vi "BaseConfigure.vi"(8 "error in (no error)":errorcluster, 11 "ChromaAcLoad in":refnum<class "ChromaAcLoad.lvclass">) -> (0 "error out":errorcluster, 3 "ChromaAcLoad out":refnum<class "ChromaAcLoad.lvclass">)   [LabVIEW 2014, in "AcPwrPlugins.lvlib" / "ChromaAcLoad.lvclass"]
uses:
  ChromaAcLoad.lvclass
  AcPwrBaseClass/AcPwrBase.lvclass/AcPwrBase.ctl
  ChromaAcLoad.lvclass/ChromaAcLoad.ctl
  AcPwrBaseClass/Accessors/Read BaseConfig.vi
  Accessors/Read Loads.vi
  AcPwrBaseClass/Accessors/Write BaseConfig.vi
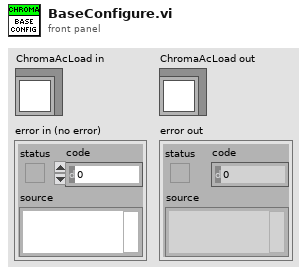
[diagram p1: front panel]
types:
  T1 = typedef "AcPwrPlugins.lvlib/AcPwrBase.lvclass/BaseConfig.ctl" = cluster{"Frequency":dbl, "FrequencyRange":dbl[], "Phases":T2[]}
  T2 = typedef "AcPwrPlugins.lvlib/AcPwrBase.lvclass/Phase.ctl" = cluster{"Enabled":bool, "VoltageLevel":dbl, "Waveform":string, "Name":string, "VoltageRange":dbl[], "CurrentLimit":dbl, "Handle":string, "Connected":bool}
  T3 = typedef "AcPwrPlugins.lvlib/ChromaAcLoad.lvclass/Load.ctl" = cluster{"AC/DC":bool, "Mode":enum16{"CC", "CP", "CR", "CV", "RLC", "RLC CP", "Inrush", "Rectified"}, "LC":cluster{"Capacitance":dbl, "Inductance":dbl, "RL":dbl, "RS":dbl}, "Resistance":dbl, "LoadSettings":T4, "Wave":enum16{""}, "LineSync":bool, "LoadShortCircuited":bool, "Slew":cluster{"RiseSlewRate":dbl, "FallSlewRate":dbl}, "Timing":cluster{"TimingOn":enum16{""}, "Hours":u32, "Minutes":u32, "Seconds":dbl, "CutoffVoltage":dbl}}
  T4 = typedef "AcPwrPlugins.lvlib/ChromaAcLoad.lvclass/LoadSettings.ctl" = cluster{"CrestFactor":dbl, "PowerFactor":dbl, "PowerLoading":dbl, "IpeakMax":dbl, "Priority":enum16{"Off", "Hold Up", "Transfer"}}
  T5 = enum16{"CC", "CP", "CR", "CV", "RLC", "RLC CP", "Inrush", "Rectified"}
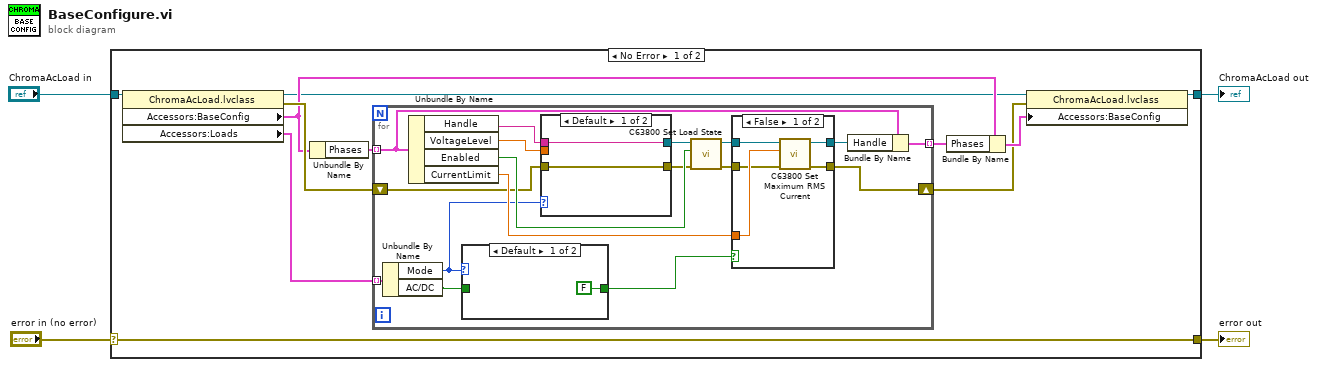
[diagram p0: block diagram]
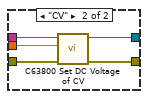
[diagram p2: hidden frame]
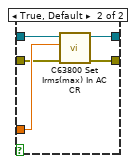
[diagram p3: hidden frame]
diagram:
  n1 = case shown="No Error" "error in (no error)" {
    selector: "error in (no error)" -> [w12 w52]
    tunnel: "ChromaAcLoad in" -> [w15 w53]
    tunnel: [w8 w53] -> w3
    tunnel: [w12 w52] -> w1
    frame No Error {
      n2 = property class="ChromaAcLoad.lvclass"(reference=w15) -> (reference out=w7:refnum<class "ChromaAcLoad.lvclass">, error out=w13:errorcluster, "Accessors:BaseConfig"=w10:T1, "Accessors:Loads"=w11:T3[])  [unwired: 1 in]
      n3 = Unbundle By Name(w10) -> ("Phases"=w14:T2[])
      n4 = for {
        tunnel: w14 -> [w25] mode=indexing
        tunnel: w11 -> [w31] mode=indexing
        tunnel: [w24] -> w9 mode=indexing
        shift-right: [w22] -> w5
        shift-left: w13 -> [w19]
        n5 = Unbundle By Name(w31) -> ("Mode"=w21:T5, "AC/DC"=w30:bool)
        n6 = Unbundle By Name(w25) -> ("Handle"=w20:string, "VoltageLevel"=w16:dbl, "Enabled"=w32:bool, "CurrentLimit"=w27:dbl)
        n7 = case shown="Default" w21 {
          tunnel: w30 -> [_ w51]
          tunnel: [FALSE ("AC/DC") w51] -> w29
          frame Default {
          }
          frame "CR" {
          }
        }
        n8 = case shown="Default" w21 {
          tunnel: w20 -> [w34 w39]
          tunnel: w19 -> [w33 w38]
          tunnel: [w34 w37] -> w18
          tunnel: [w33 w36] -> w17
          tunnel: w16 -> [_ w35]
          frame Default {
          }
          frame "CV" {
            n9 = call <instrlib>:"C63800 Set DC Voltage of CV.vi"("error in (no error)"=w38, "SetDCVoltageofCV"=w35, "Instrument Handle"=w39) -> ("error out"=w36:errorcluster, "Instrument Handle out"=w37:refnum<k15>)  [unwired: 7 in]
          }
        }
        n10 = call <instrlib>:"C63800 Set Load State.vi"("error in (no error)"=w17, "Load State"=w32, "Instrument Handle"=w18) -> ("error out"=w26:errorcluster, "Instrument Handle out"=w28:refnum<k15>)  [unwired: 7 in]
        n11 = case shown="False" w29 {
          tunnel: w28 -> [w44 w49]
          tunnel: w27 -> [w43 w48]
          tunnel: w26 -> [w42 w47]
          tunnel: [w41 w46] -> w23
          tunnel: [w40 w45] -> w22
          frame False {
            n12 = call <instrlib>:"C63800 Set Maximum RMS Current.vi"("error in (no error)"=w42, "Set Max RMS Current"=w43, "Instrument Handle"=w44) -> ("error out"=w40:errorcluster, "Instrument Handle out"=w41:refnum<k15>)  [unwired: 7 in]
          }
          frame True, Default {
            n13 = call <instrlib>:"C63800 Set Irms(max) In AC CR.vi"("error in (no error)"=w47, "I_max"=w48, "Instrument Handle"=w49) -> ("error out"=w45:errorcluster, "Instrument Handle out"=w46:refnum<k15>)  [unwired: 7 in]
          }
        }
        n14 = Bundle By Name(cluster=w25, "Handle"=w23) -> (w24:T2)
      }
      n15 = Bundle By Name(cluster=w10, "Phases"=w9) -> (w6:T1)
      n16 = property class="ChromaAcLoad.lvclass"(reference=w7, error in=w5, "Accessors:BaseConfig"=w6) -> (reference out=w8:refnum<class "ChromaAcLoad.lvclass">)  [unwired: 1 out]
    }
    frame Error {
    }
  }
  "error out" <- w1
  "ChromaAcLoad out" <- w3
